vi "Write ASCII Char.vi"(8 "error in (no error)":errorcluster, 9 "Char":string, 11 "Grove I2C Matrix LED Driver in":refnum<class "Grove I2C Matrix LED Driver.lvclass">) -> (0 "error out":errorcluster, 3 "Grove I2C Matrix LED Driver out":refnum<class "Grove I2C Matrix LED Driver.lvclass">)   [LabVIEW 2020, in "CTI-Peripheral.lvlib" / "Grove I2C Matrix LED Driver.lvclass"]
uses:
  Grove I2C Matrix LED Driver.lvclass
  Grove I2C Matrix LED Driver.lvclass/Grove I2C Matrix LED Driver.ctl
  CTI/I2C Connection/I2C Connection.lvclass/I2C Connection.ctl
  CTI/Session/I2C Write Data.vi
  CTI/I2C Connection/I2C Connection.lvclass
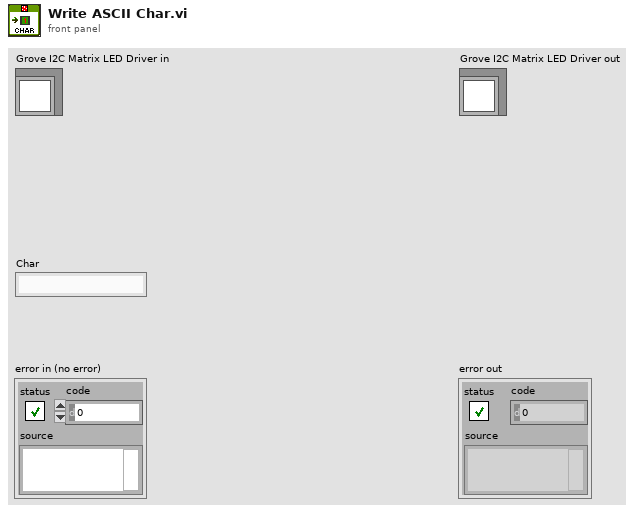
[diagram p1: front panel]
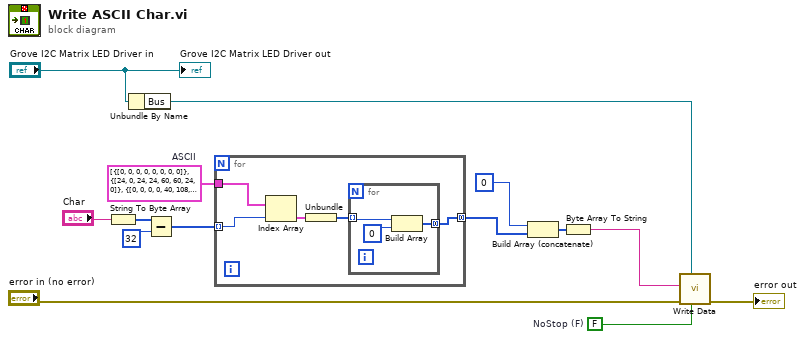
[diagram p0: block diagram]
diagram:
  w7 = FALSE  # NoStop (F)
  w11 = cluster{"BytesOut":u8[]}[] [{"BytesOut"=[0, 0, 0, 0, 0, 0, 0, 0]}, {"BytesOut"=[24, 0, 24, 24, 60, 60, 24, 0]}, {"BytesOut"=[0, 0, 0, 0, 40, 108, 108, 0]}, {"BytesOut"=[108, 108, 254, 108, 254, 108, 108, 0]}, {"BytesOut"=[16, 60, 64, 56, 4, 120, 16, 0]}, {"BytesOut"=[96, 102, 12, 24, 48, 102, 6, 0]}, {"BytesOut"=[252, 102, 166, 20, 60, 102, 60, 0]}, {"BytesOut"=[0, 0, 0, 12, 24, 24, 24, 0]}, {"BytesOut"=[96, 48, 24, 24, 24, 48, 96, 0]}, {"BytesOut"=[6, 12, 24, 24, 24, 12, 6, 0]}, {"BytesOut"=[0, 108, 56, 254, 56, 108, 0, 0]}, {"BytesOut"=[0, 16, 16, 124, 16, 16, 0, 0]}, {"BytesOut"=[6, 12, 12, 12, 0, 0, 0, 0]}, {"BytesOut"=[0, 0, 0, 60, 0, 0, 0, 0]}, {"BytesOut"=[6, 6, 0, 0, 0, 0, 0, 0]}, {"BytesOut"=[0, 6, 12, 24, 48, 96, 0, 0]}, {"BytesOut"=[28, 34, 34, 34, 34, 34, 34, 28]}, {"BytesOut"=[28, 8, 8, 8, 8, 8, 12, 8]}, {"BytesOut"=[62, 4, 8, 16, 32, 32, 34, 28]}, {"BytesOut"=[28, 34, 32, 32, 24, 32, 34, 28]}, {"BytesOut"=[32, 32, 62, 34, 36, 40, 48, 32]}, {"BytesOut"=[28, 34, 32, 32, 30, 2, 2, 62]}, {"BytesOut"=[28, 34, 34, 34, 30, 2, 34, 28]}, {"BytesOut"=[4, 4, 4, 8, 16, 32, 32, 62]}, {"BytesOut"=[28, 34, 34, 34, 28, 34, 34, 28]}, {"BytesOut"=[28, 34, 32, 60, 34, 34, 34, 28]}, {"BytesOut"=[0, 24, 24, 0, 24, 24, 0, 0]}, {"BytesOut"=[12, 24, 24, 0, 24, 24, 0, 0]}, {"BytesOut"=[96, 48, 24, 12, 24, 48, 96, 0]}, {"BytesOut"=[0, 0, 60, 0, 60, 0, 0, 0]}, {"BytesOut"=[6, 12, 24, 48, 24, 12, 6, 0]}, {"BytesOut"=[24, 0, 24, 56, 96, 102, 60, 0]}, {"BytesOut"=[0, 60, 66, 26, 58, 34, 28, 0]}, {"BytesOut"=[0, 51, 51, 63, 51, 51, 30, 12]}, {"BytesOut"=[0, 63, 102, 102, 62, 102, 102, 63]}, {"BytesOut"=[0, 60, 102, 3, 3, 3, 102, 60]}, {"BytesOut"=[0, 31, 54, 102, 102, 102, 54, 31]}, {"BytesOut"=[0, 127, 70, 22, 30, 22, 70, 127]}, {"BytesOut"=[0, 15, 6, 22, 30, 22, 70, 127]}, {"BytesOut"=[0, 124, 102, 115, 3, 3, 102, 60]}, {"BytesOut"=[0, 51, 51, 51, 63, 51, 51, 51]}, {"BytesOut"=[0, 30, 12, 12, 12, 12, 12, 30]}, {"BytesOut"=[0, 30, 51, 51, 48, 48, 48, 120]}, {"BytesOut"=[0, 103, 102, 54, 30, 54, 102, 103]}, {"BytesOut"=[0, 127, 102, 70, 6, 6, 6, 15]}, {"BytesOut"=[0, 99, 99, 107, 127, 127, 119, 99]}, {"BytesOut"=[0, 99, 99, 115, 123, 111, 103, 99]}, {"BytesOut"=[0, 28, 54, 99, 99, 99, 54, 28]}, {"BytesOut"=[0, 15, 6, 6, 62, 102, 102, 63]}, {"BytesOut"=[0, 56, 30, 59, 51, 51, 51, 30]}, {"BytesOut"=[0, 103, 102, 54, 62, 102, 102, 63]}, {"BytesOut"=[0, 30, 51, 56, 14, 7, 51, 30]}, {"BytesOut"=[0, 30, 12, 12, 12, 12, 45, 63]}, {"BytesOut"=[0, 63, 51, 51, 51, 51, 51, 51]}, {"BytesOut"=[0, 12, 30, 51, 51, 51, 51, 51]}, {"BytesOut"=[0, 99, 119, 127, 107, 99, 99, 99]}, {"BytesOut"=[0, 99, 54, 28, 28, 54, 99, 99]}, {"BytesOut"=[0, 30, 12, 12, 30, 51, 51, 51]}, {"BytesOut"=[0, 127, 102, 76, 24, 49, 99, 127]}, {"BytesOut"=[120, 24, 24, 24, 24, 24, 120, 0]}, {"BytesOut"=[0, 96, 48, 24, 12, 6, 0, 0]}, {"BytesOut"=[30, 24, 24, 24, 24, 24, 30, 0]}, {"BytesOut"=[0, 0, 0, 130, 68, 40, 16, 0]}, {"BytesOut"=[126, 0, 0, 0, 0, 0, 0, 0]}, {"BytesOut"=[0, 0, 0, 0, 96, 48, 48, 0]}, {"BytesOut"=[0, 110, 51, 62, 48, 30, 0, 0]}, {"BytesOut"=[0, 59, 102, 102, 62, 6, 6, 7]}, {"BytesOut"=[0, 30, 51, 3, 51, 30, 0, 0]}, {"BytesOut"=[0, 110, 51, 51, 62, 48, 48, 56]}, {"BytesOut"=[0, 30, 3, 63, 51, 30, 0, 0]}, {"BytesOut"=[0, 15, 6, 6, 15, 6, 54, 28]}, {"BytesOut"=[31, 48, 62, 51, 51, 110, 0, 0]}, {"BytesOut"=[0, 103, 102, 102, 110, 54, 6, 7]}, {"BytesOut"=[0, 30, 12, 12, 12, 14, 0, 12]}, {"BytesOut"=[30, 51, 51, 48, 48, 48, 0, 48]}, {"BytesOut"=[0, 103, 54, 30, 54, 102, 6, 7]}, {"BytesOut"=[0, 30, 12, 12, 12, 12, 12, 14]}, {"BytesOut"=[0, 99, 107, 127, 127, 51, 0, 0]}, {"BytesOut"=[0, 51, 51, 51, 51, 31, 0, 0]}, {"BytesOut"=[0, 30, 51, 51, 51, 30, 0, 0]}, {"BytesOut"=[15, 6, 62, 102, 102, 59, 0, 0]}, {"BytesOut"=[120, 48, 62, 51, 51, 110, 0, 0]}, {"BytesOut"=[0, 15, 6, 102, 110, 59, 0, 0]}, {"BytesOut"=[0, 31, 48, 30, 3, 62, 0, 0]}, {"BytesOut"=[0, 24, 44, 12, 12, 62, 12, 8]}, {"BytesOut"=[0, 110, 51, 51, 51, 51, 0, 0]}, {"BytesOut"=[0, 12, 30, 51, 51, 51, 0, 0]}, {"BytesOut"=[0, 54, 127, 127, 107, 99, 0, 0]}, {"BytesOut"=[0, 99, 54, 28, 54, 99, 0, 0]}, {"BytesOut"=[31, 48, 62, 51, 51, 51, 0, 0]}, {"BytesOut"=[0, 63, 38, 12, 25, 63, 0, 0]}, {"BytesOut"=[112, 24, 24, 12, 24, 24, 112, 0]}, {"BytesOut"=[0, 8, 8, 8, 8, 8, 8, 0]}, {"BytesOut"=[14, 24, 24, 48, 24, 24, 14, 0]}, {"BytesOut"=[0, 0, 0, 54, 92, 0, 0, 0, 0, 0, 0, 0, 0]}]  # ASCII
  n1 = String To Byte Array(string="Char") -> (unsigned byte array=w14:u8[])
  n2 = Unbundle By Name("Grove I2C Matrix LED Driver in") -> ("Bus"=w1:refnum<class "I2C Connection.lvclass">)
  n3 = Subtract(x=w14, y=32) -> (x-y=w10:i32[])
  n4 = for {
    tunnel: w11 -> [w18]
    tunnel: w10 -> [w17] mode=indexing
    tunnel: [w15] -> w2 mode=concatenating
    n5 = Index Array(array=w18, index=w17) -> (element=w19:cluster{"BytesOut":u8[]})
    n6 = Unbundle(w19) -> ("BytesOut"=w16:u8[])
    n7 = for {
      tunnel: w16 -> [w22] mode=indexing
      tunnel: [w20] -> w15 mode=concatenating
      n8 = Build Array(w22, u8 0 ("Value")) -> (w20:u8[])
    }
  }
  n9 = Build Array (concatenate)(u8 0 ("Value"), w2) -> (w9:u8[])
  n10 = Byte Array To String(unsigned byte array=w9) -> (string=w6:string)
  n11 = call "Write Data.vi"("NoStop (F)"=w7, "I2C Connection"=w1, "error in (no error)"="error in (no error)", "Data"=w6) -> ("error out"=→"error out":errorcluster)  [unwired: 7 in]
  "Grove I2C Matrix LED Driver out" <- "Grove I2C Matrix LED Driver in"
